vi "Create Constants.vi"(9 "Z":dbl, 10 "Y":dbl, 11 "X":dbl) -> (3 "constants cluster":cluster{"a":dbl, "b":dbl, "c":dbl, "d":dbl})   [LabVIEW 2016]
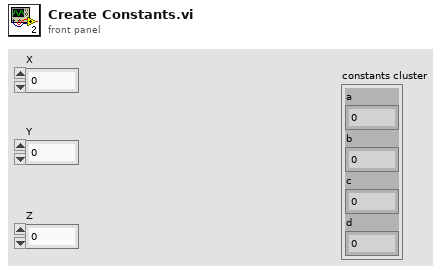
[diagram p1: front panel]
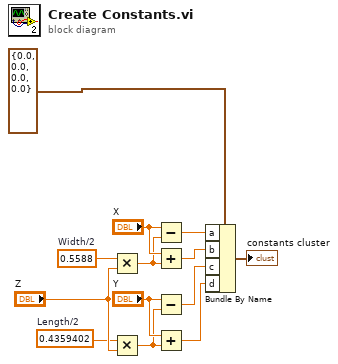
[diagram p0: block diagram]
diagram:
  w7 = 0.4359402  # Length/2
  w9 = 0.5588  # Width/2
  n1 = Multiply(x=w9, y="Z") -> (x*y=w2:dbl)
  n2 = Multiply(x=w7, y="Z") -> (x*y=w4:dbl)
  n3 = Subtract(x="X", y=w2) -> (x-y=w11:dbl)
  n4 = Add(x="X", y=w2) -> (x+y=w8:dbl)
  n5 = Subtract(x="Y", y=w4) -> (x-y=w6:dbl)
  n6 = Add(x="Y", y=w4) -> (x+y=w3:dbl)
  n7 = Bundle By Name(cluster=cluster{"d":dbl, "c":dbl, "b":dbl, "a":dbl} {"d"=0.0, "c"=0.0, "b"=0.0, "a"=0.0}, "a"=w11, "b"=w8, "c"=w6, "d"=w3) -> (→"constants cluster":cluster{"d":dbl, "c":dbl, "b":dbl, "a":dbl})
